vi "increasedNumber.vi"(11 "increase?":bool) -> (3 "increased n":u32)   [LabVIEW 2017]
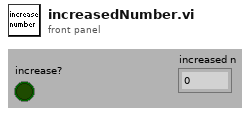
[diagram p1: front panel]
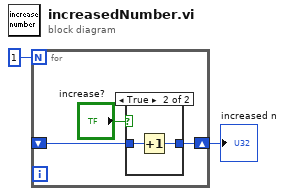
[diagram p0: block diagram]
diagram:
  n1 = for {
    N: 1 -> [_]
    shift-right: [w3] -> w1
    shift-left: _ -> [w4]
    n2 = case shown="True" "increase?" {
      tunnel: w4 -> [w6 w8]
      tunnel: [w6 w7] -> w3
      frame False {
      }
      frame True {
        n3 = Increment ("加1")(x=w8) -> (x+1=w7:u32)
      }
    }
  }
  "increased n" <- w1
